vi "Read Ack Time.vi"(8 "error in (no error)":errorcluster, 11 "AE in":refnum<class "AE.lvclass">) -> (0 "error out":errorcluster, 2 "Ack Time":timestamp, 3 "AE out":refnum<class "AE.lvclass">)   [LabVIEW 2013, in "CS++ProcessVariables.lvlib" / "AE.lvclass"]
uses:
  AE.lvclass
  AE.lvclass/AE.ctl
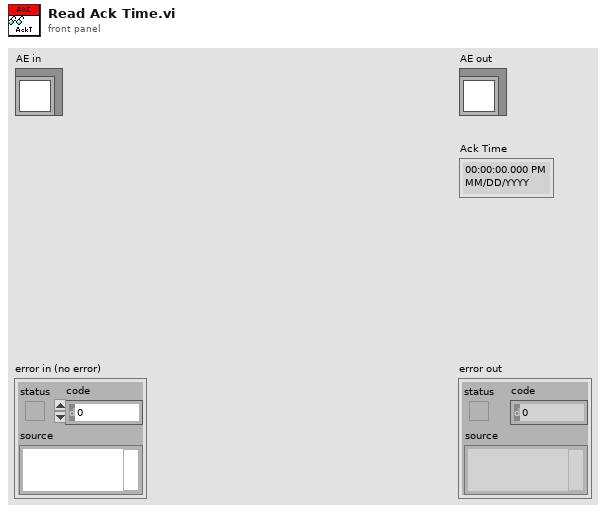
[diagram p1: front panel]
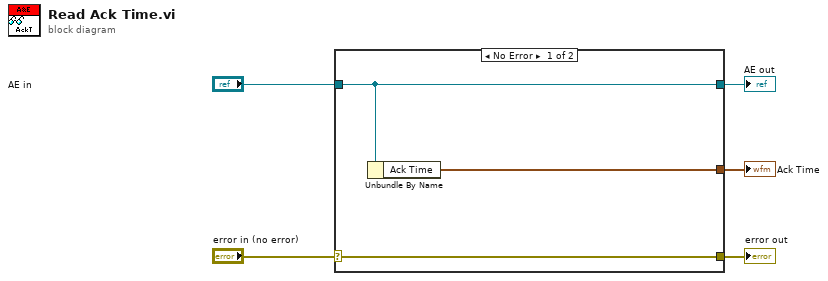
[diagram p0: block diagram]
diagram:
  n1 = case shown="No Error" "error in (no error)" {
    selector: "error in (no error)" -> [w8 w9]
    tunnel: [w8 w9] -> w4
    tunnel: [w7 w10] -> w2
    tunnel: "AE in" -> [w7 w10]
    tunnel: [w6 _] -> w1
    frame No Error {
      n2 = Unbundle By Name(w7) -> ("Ack Time"=w6:timestamp)
    }
    frame Error {
    }
  }
  "error out" <- w4
  "AE out" <- w2
  "Ack Time" <- w1
